vi "sortByChannel.vi"(8 "error in (no error)":errorcluster, 10 "Array":T2(array[cluster]) {"times" format="%_18g"}, 11 "ScriptEventList in":refnum<class "ScriptEventList.lvclass">) -> (0 "error out":errorcluster, 2 "data":T1(array[cluster]), 3 "ScriptEventList out":refnum<class "ScriptEventList.lvclass">)   [LabVIEW 2011, in "Tools.lvlib" / "Scripting.lvlib" / "ScriptEventList.lvclass"]
uses:
  ScriptEventList.lvclass
  DatabaseHelpers/Database Objects/Channel/Channel.lvclass
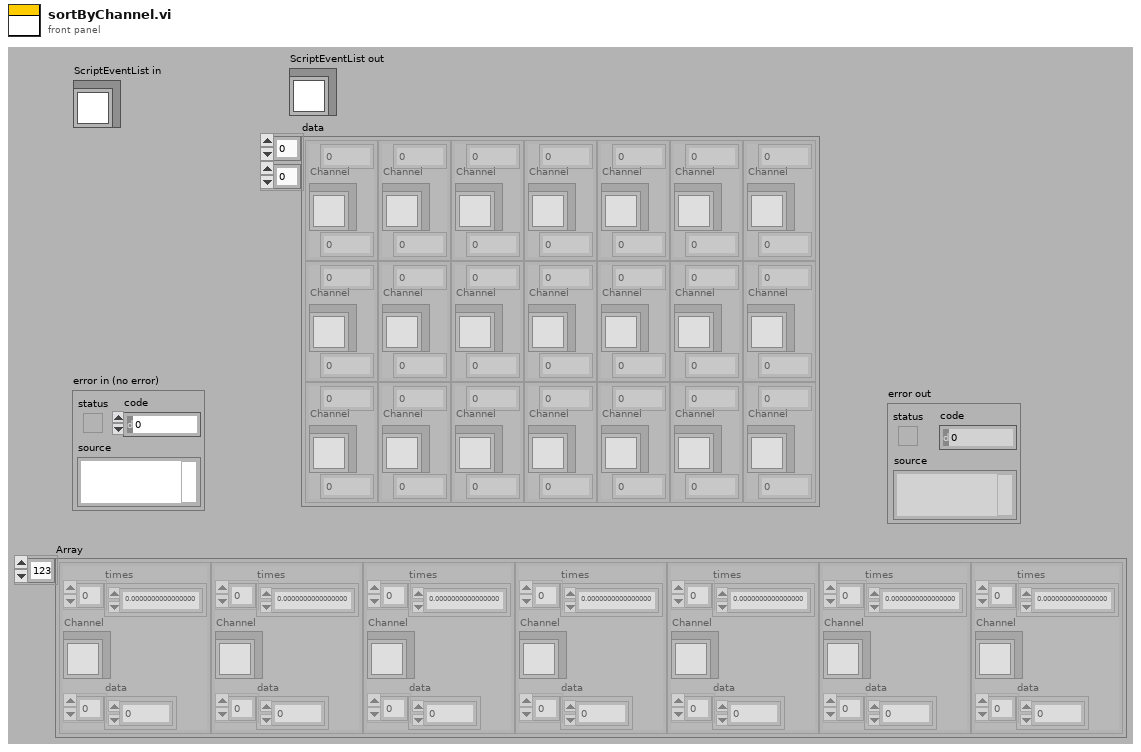
[diagram p1: front panel]
types:
  T1 = cluster{dbl, "Channel":refnum<class "Channel.lvclass">, dbl}[][]
  T2 = cluster{"times":dbl[], "Channel":refnum<class "Channel.lvclass">, "data":dbl[]}[]
  T3 = cluster{"times":dbl[], "Channel":refnum<class "Channel.lvclass">, "data":dbl[]}
  T4 = cluster{dbl, "Channel":refnum<class "Channel.lvclass">, dbl}
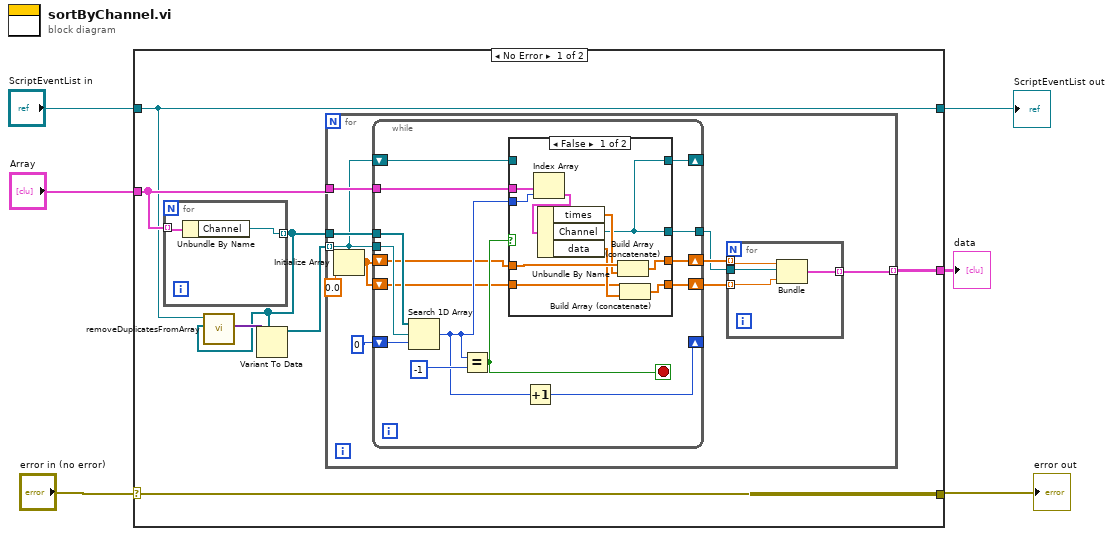
[diagram p0: block diagram]
diagram:
  n1 = case shown="No Error" "error in (no error)" {
    selector: "error in (no error)" -> [w13 w59]
    tunnel: [w13 w59] -> w5
    tunnel: [w8 w58] -> w3
    tunnel: "ScriptEventList in" -> [w8 w58]
    tunnel: "Array" -> [w12 _]
    tunnel: [w7 _] -> w1
    frame No Error {
      n2 = for {
        tunnel: w12 -> [w57] mode=indexing
        tunnel: [w56] -> w9 mode=indexing
        n3 = Unbundle By Name(w57) -> ("Channel"=w56:refnum<class "Channel.lvclass">)
      }
      n4 = call "removeDuplicatesFromArray.vi"("Array"=w9, "ScriptEventList in"=w8) -> ("Array out"=w11:variant[])  [unwired: 7 in, 2 out]
      n5 = Variant To Data(type=w9, Variant=w11) -> (data=w10:refnum<class "Channel.lvclass">[])  [unwired: 1 in, 1 out]
      n6 = for {
        tunnel: w12 -> [w21]
        tunnel: w9 -> [w23]
        tunnel: w10 -> [w14] mode=indexing
        tunnel: [w15] -> w7 mode=indexing
        n7 = Initialize Array(0.0) -> (w19:dbl[])  [unwired: 1 in]
        n8 = while {
          tunnel: w23 -> [w42]
          tunnel: w21 -> [w38]
          tunnel: w14 -> [w41]
          shift-right: [w36] -> _
          shift-left: 0 -> [w37]
          shift-right: [w34] -> w18
          shift-left: w19 -> [w33]
          shift-right: [w32] -> w17
          shift-left: w19 -> [w31]
          tunnel: [w30] -> w16
          shift-right: [w29] -> _
          shift-left: w14 -> [w28]
          stop <- w39 stop-if-true
          n9 = Search 1D Array(1D array=w42, element=w41, start index (0)=w37) -> (index of element=w35:i32)
          n10 = Equal?(x=w35, y=-1) -> (x = y?=w39:bool)
          n11 = case shown="False" w39 {
            tunnel: w38 -> [w52 _]
            tunnel: w35 -> [w51 _]
            tunnel: [w49 w55] -> w34
            tunnel: w33 -> [w48 w55]
            tunnel: [w45 w54] -> w32
            tunnel: w31 -> [w44 w54]
            tunnel: [w43 w53] -> w30
            tunnel: [w43 w53] -> w29
            tunnel: w28 -> [_ w53]
            frame False {
              n12 = Index Array(array=w52, index=w51) -> (element=w50:T3)
              n13 = Unbundle By Name(w50) -> ("times"=w47:dbl[], "Channel"=w43:refnum<class "Channel.lvclass">, "data"=w46:dbl[])
              n14 = Build Array (concatenate)(w48, w47) -> (w49:dbl[])
              n15 = Build Array (concatenate)(w44, w46) -> (w45:dbl[])
            }
            frame True {
            }
          }
          n16 = Increment(x=w35) -> (x+1=w36:i32)
        }
        n17 = for {
          tunnel: w18 -> [w27] mode=indexing
          tunnel: w17 -> [w25] mode=indexing
          tunnel: w16 -> [w26]
          tunnel: [w24] -> w15 mode=indexing
          n18 = Bundle(w27, "Channel"=w26, w25) -> (w24:T4)  [unwired: 1 in]
        }
      }
    }
    frame Error {
    }
  }
  "error out" <- w5
  "ScriptEventList out" <- w3
  "data" <- w1
